vi "Replace Empty String.vi"(10 "replacement string":string, 11 "string in":string) -> (3 "string out":string)   [LabVIEW 2014, in "vipm-to-nipm-package-converter.lvlib"]
doc: "If incoming string is an empty string, this VI will replace it with the specified replacement string"
uses:
  vipm-to-nipm-package-converter.lvlib
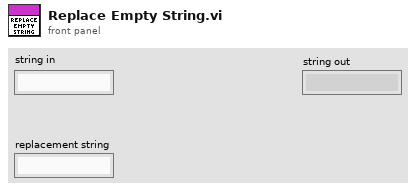
[diagram p1: front panel]
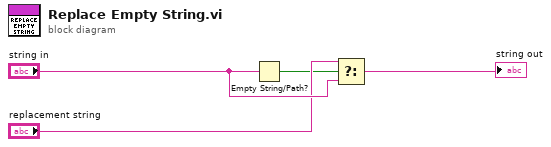
[diagram p0: block diagram]
diagram:
  n1 = Empty String/Path?(string/path="string in") -> (empty?=w1:bool)
  n2 = Select(t="replacement string", s=w1, f="string in") -> (s? t:f=→"string out":string)
